vi "Read Channel names.vi"(8 "error in (no error)":errorcluster, 11 "DAQmx Digitizer in":refnum<class "DAQmx Digitizer.lvclass">) -> (0 "error out":errorcluster, 2 "Channel names":string[](array[string]), 3 "DAQmx Digitizer out":refnum<class "DAQmx Digitizer.lvclass">)   [LabVIEW 2015, in "DAQmx Digitizer.lvclass"]
uses:
  DAQmx Digitizer.lvclass
  DAQmx Digitizer.lvclass/DAQmx Digitizer.ctl
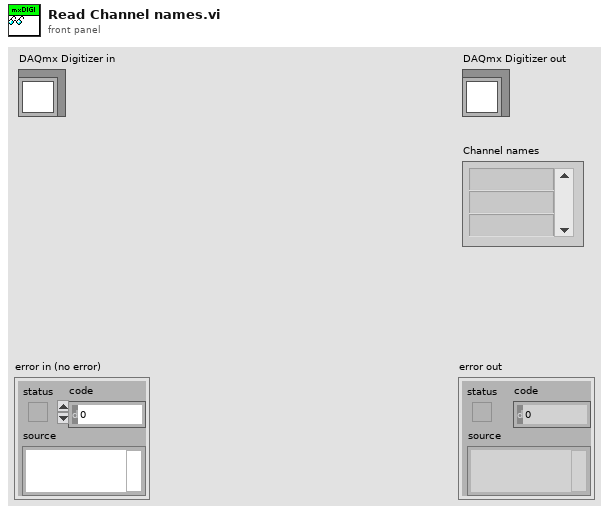
[diagram p1: front panel]
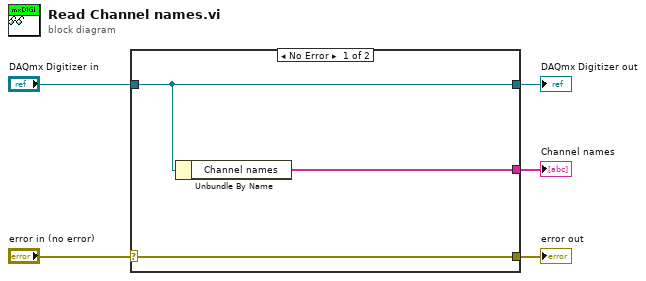
[diagram p0: block diagram]
diagram:
  n1 = case shown="No Error" "error in (no error)" {
    selector: "error in (no error)" -> [w8 w9]
    tunnel: [w8 w9] -> w4
    tunnel: [w7 w10] -> w2
    tunnel: "DAQmx Digitizer in" -> [w7 w10]
    tunnel: [w6 _] -> w1
    frame No Error {
      n2 = Unbundle By Name(w7) -> ("Channel names"=w6:string[])
    }
    frame Error {
    }
  }
  "error out" <- w4
  "DAQmx Digitizer out" <- w2
  "Channel names" <- w1
